vi "Administration Tasks.vi"(8 "error in (no error)":errorcluster) -> (0 "error out":errorcluster, 3 "Message":string)   [LabVIEW 2014]
uses:
  controls/UI Trainers.ctl
  controls/UI Pass Types.ctl
  controls/UI Statistics.ctl
  controls/UI Languages.ctl
  controls/UI Date Time.ctl
panel:
  out "date/time string":string
  in  "Help":bool
  in  "Reset":bool
  in  "Back":bool
  in  "Date Time":T1
  in  "Languages":T2
  in  "Statistics":T3
  in  "Pass Types":T4
  in  "Trainers":T5
  # "Administration Tasks"
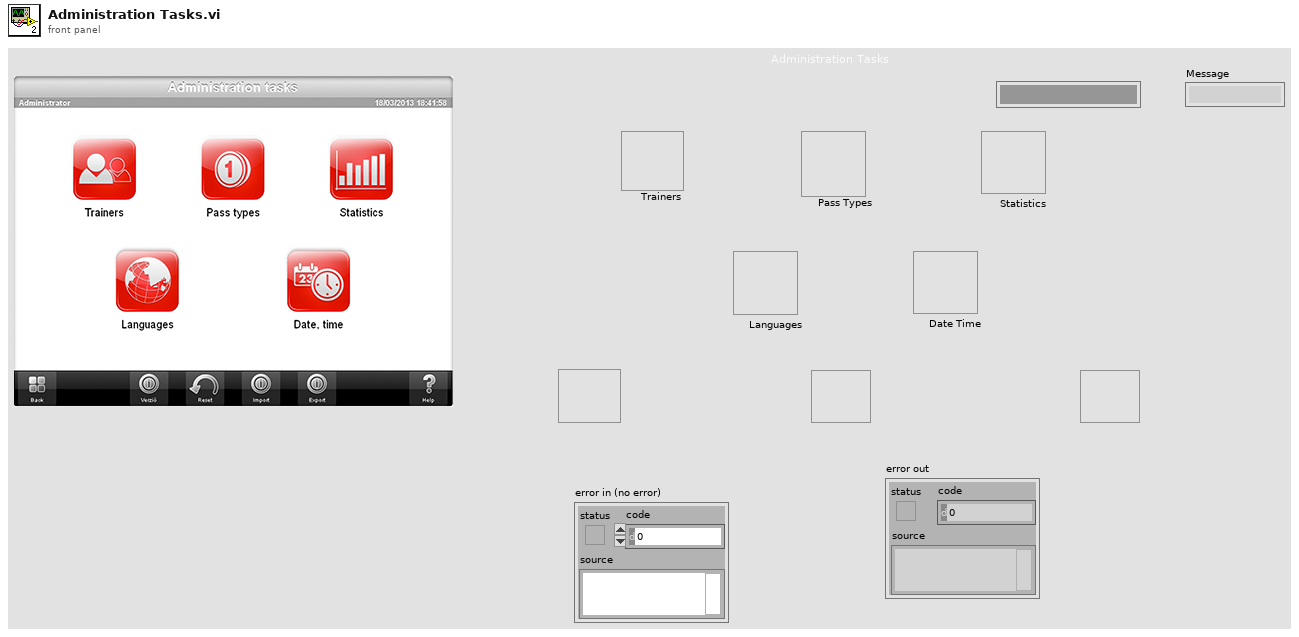
[diagram p1: front panel]
types:
  T1 = typedef "UI Date Time.ctl" = bool
  T2 = typedef "UI Languages.ctl" = bool
  T3 = typedef "UI Statistics.ctl" = bool
  T4 = typedef "UI Pass Types.ctl" = bool
  T5 = typedef "UI Trainers.ctl" = bool
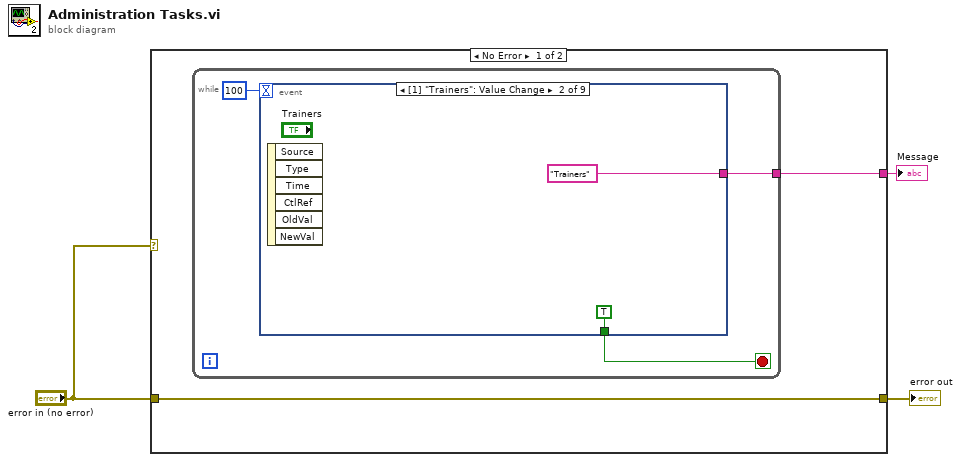
[diagram p0: block diagram]
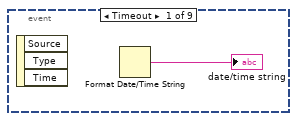
[diagram p2: hidden frame]
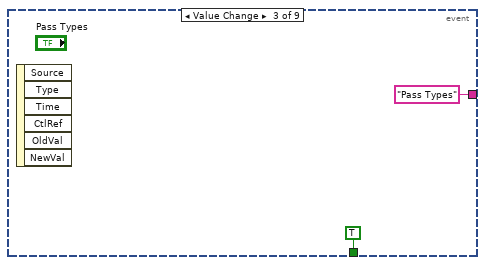
[diagram p3: hidden frame]
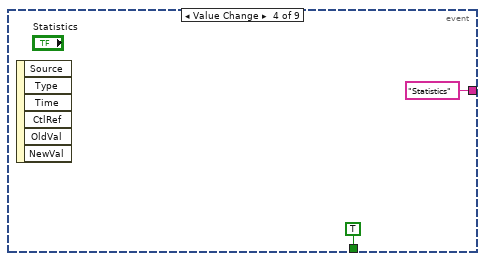
[diagram p4: hidden frame]
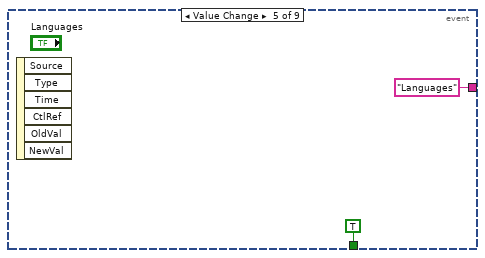
[diagram p5: hidden frame]
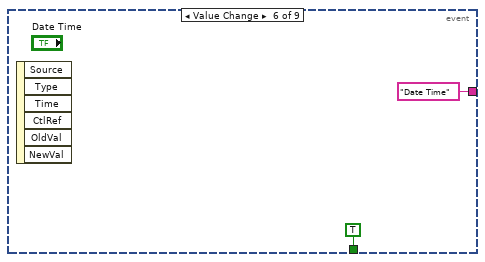
[diagram p6: hidden frame]
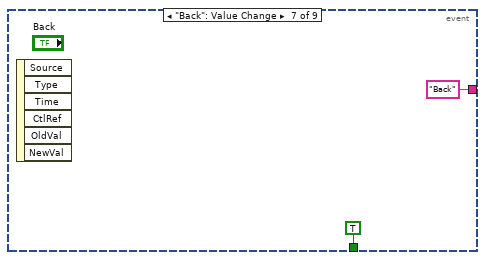
[diagram p7: hidden frame]
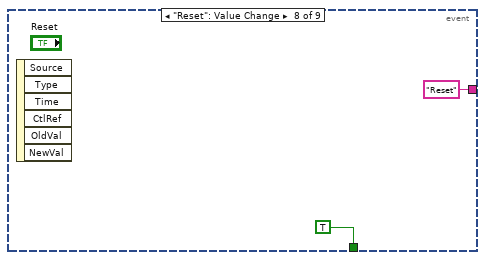
[diagram p8: hidden frame]
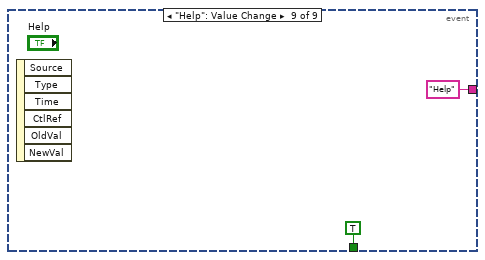
[diagram p9: hidden frame]
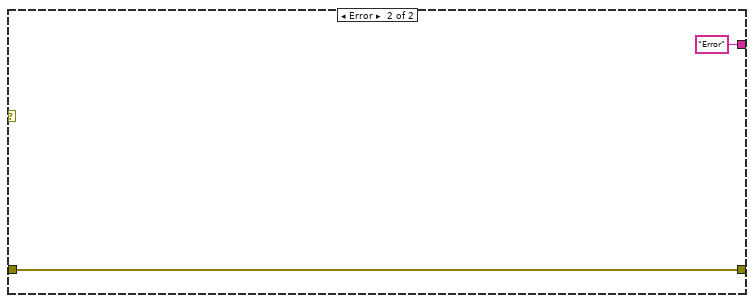
[diagram p10: hidden frame]
diagram:
  n1 = case shown="No Error" "error in (no error)" {
    tunnel: "error in (no error)" -> [w5 w27]
    tunnel: [w5 w27] -> w2
    tunnel: [w4 "Error" ("Message")] -> w1
    frame No Error {
      n2 = while {
        tunnel: [w6] -> w4
        stop <- w8 stop-if-true
        n3 = event shown="[1] \"Trainers\": Value Change" {
          selector: _ -> [_ _ _ _ _ _ _ _ _]
          dyn-events: _ -> [_ _ _ _ _ _ _ _ _]
          timeout: 100 -> [_ _ _ _ _ _ _ _ _]
          tunnel: [_ TRUE TRUE TRUE TRUE TRUE TRUE TRUE TRUE] -> w8
          tunnel: [_ "Trainers" ("Message") "Pass Types" ("Message") "Statistics" ("Message") "Languages" ("Message") "Date Time" ("Message") "Back" ("Message") "Reset" ("Message") "Help" ("Message")] -> w6
          event Timeout {
            n4 = event-data() -> ()  [unwired: 1 in, 3 out]
            n5 = Format Date/Time String() -> (date/time string=→"date/time string":string)  [unwired: 3 in]
          }
          event Value Change {
            n6 = event-data() -> ()  [unwired: 1 in, 6 out]
          }
          event Value Change {
            n7 = event-data() -> ()  [unwired: 1 in, 6 out]
          }
          event Value Change {
            n8 = event-data() -> ()  [unwired: 1 in, 6 out]
          }
          event Value Change {
            n9 = event-data() -> ()  [unwired: 1 in, 6 out]
          }
          event Value Change {
            n10 = event-data() -> ()  [unwired: 1 in, 6 out]
          }
          event "Back": Value Change {
            n11 = event-data() -> ()  [unwired: 1 in, 6 out]
          }
          event "Reset": Value Change {
            n12 = event-data() -> ()  [unwired: 1 in, 6 out]
          }
          event "Help": Value Change {
            n13 = event-data() -> ()  [unwired: 1 in, 6 out]
          }
        }
      }
    }
    frame Error {
    }
  }
  "error out" <- w2
  "Message" <- w1
